vi "Set Actuator Position.vi"(8 "error in (no error)":errorcluster, 10 "Position (1 to NP)":u32=1 min=1 max=100, 11 "VISA resource name":refnum<visa-resource-name>) -> (0 "error out":errorcluster, 3 "VISA resource name out":refnum<visa-resource-name>)   [LabVIEW 2018]
doc: "Moves the actuator to the position specified, where it can be from 1 to NP (multiposition, mode 3).\nThis function should not be used for modes 1 and 2.\n\n\n(Nimble Focus Consulting 2019)"
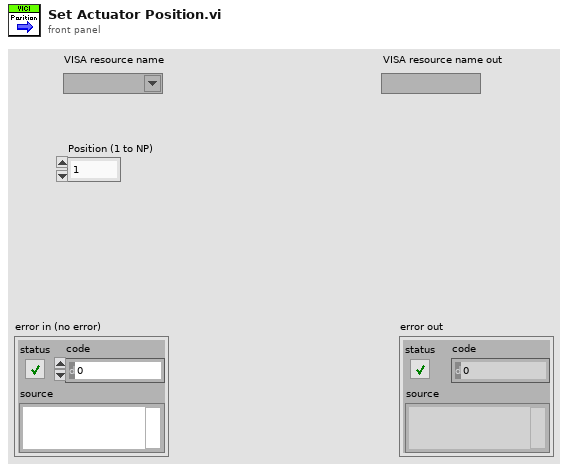
[diagram p1: front panel]
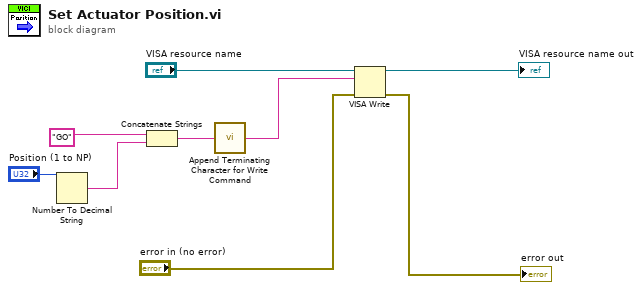
[diagram p0: block diagram]
diagram:
  n1 = Number To Decimal String(number="Position (1 to NP)") -> (decimal integer string=w2:string)  [unwired: 1 in]
  n2 = Concatenate Strings("GO" ("Command in"), w2) -> (w1:string)
  n3 = call "Append Terminating Character for Write Command.vi"("Command in"=w1) -> ("Command with Terminating character out"=w5:string)
  n4 = VISA Write(VISA resource name="VISA resource name", write buffer=w5, error in (no error)="error in (no error)") -> (VISA resource name out=→"VISA resource name out":refnum<visa-resource-name>, error out=→"error out":errorcluster)  [unwired: 1 out]
